vi "Progammable Assembly.vi"   [LabVIEW 2016]
uses:
  Classes/Controller/Controller.lvclass
  Classes/Assembly/Assembly Run.lvclass
  Classes/Routine/Routine Enum.ctl
  Classes/Routine/Routine.lvclass
  Classes/Routine/Settings.ctl
  Classes/Workspace/Fixture Enum.ctl
  Classes/Workspace/Fixture.lvclass
types:
  T1 = typedef "Routine.lvclass/Settings.ctl" = enum16{"Default", "Custom"}
  T2 = typedef "Fixture.lvclass/Fixture Enum.ctl" = enum16{"Assembly Tray", "Syringe Space", "Component", "Pick Up Tool", "Current Position"}
  T3 = typedef "Routine.lvclass/Routine Enum.ctl" = enum16{"Primary Pick Up", "Pick Up All", "Put Down Secondary", "Put Down All", "Release Syringe", "Secondary Pick Up", "Secure Syringe", "Dispense on Plate", "Dispense on Kapton", "Dispense on Sensor"}
  T4 = typedef "Controller.lvclass/Controllers.ctl" = cluster{"I-O.lvclass":refnum<class "I-O.lvclass">, "Motion.lvclass":refnum<class "Motion.lvclass">, "Dispenser.lvclass":refnum<class "Dispenser.lvclass">}
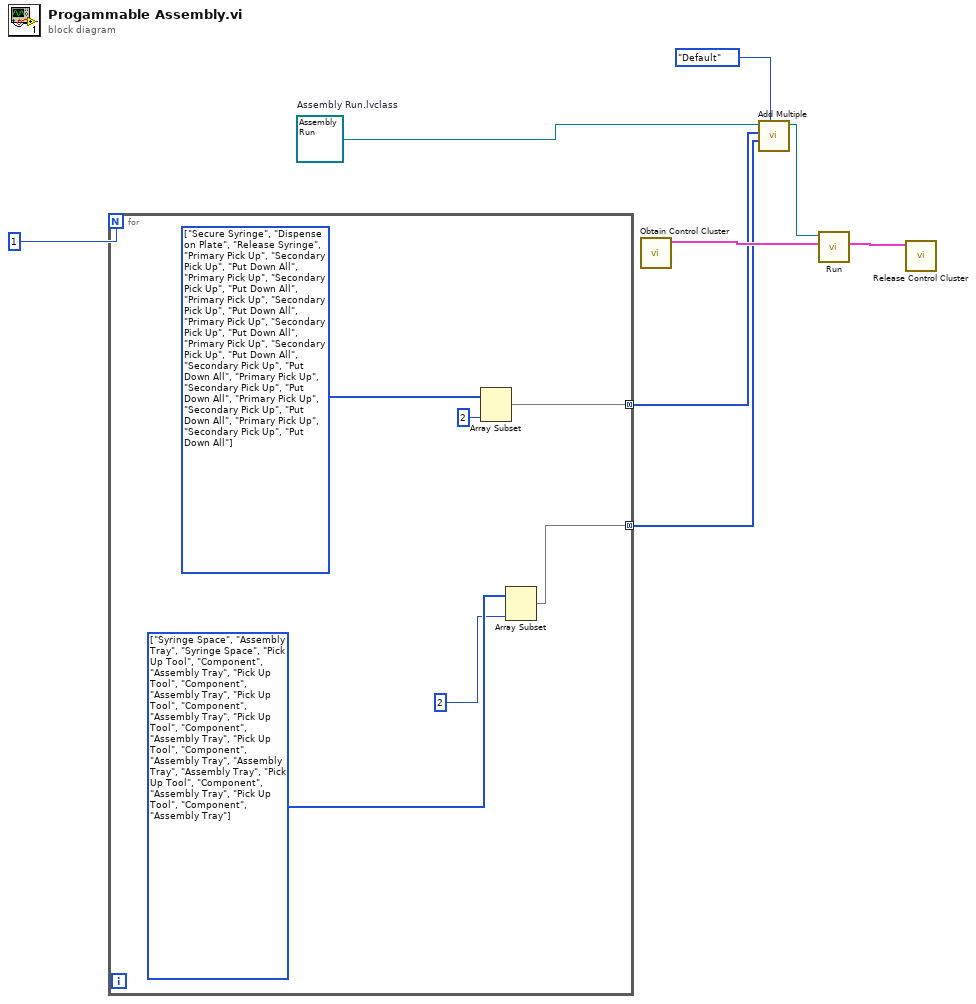
[diagram p0: block diagram]
diagram:
  w1 = refnum<class "Assembly Run.lvclass"> refnum  # Assembly Run.lvclass
  n1 = for {
    N: 1 -> [_]
    tunnel: [w13] -> w5 mode=concatenating
    tunnel: [w10] -> w2 mode=concatenating
    w11 = T2[] [enum."Syringe Space", enum."Assembly Tray", enum."Syringe Space", enum."Pick Up Tool", enum."Component", enum."Assembly Tray", enum."Pick Up Tool", enum."Component", enum."Assembly Tray", enum."Pick Up Tool", enum."Component", enum."Assembly Tray", enum."Pick Up Tool", enum."Component", enum."Assembly Tray", enum."Pick Up Tool", enum."Component", enum."Assembly Tray", enum."Assembly Tray", enum."Assembly Tray", enum."Pick Up Tool", enum."Component", enum."Assembly Tray", enum."Pick Up Tool", enum."Component", enum."Assembly Tray"] items=["Assembly Tray", "Syringe Space", "Component", "Pick Up Tool", "Current Position"]
    w14 = T3[] [enum."Secure Syringe", enum."Dispense on Plate", enum."Release Syringe", enum."Primary Pick Up", enum."Secondary Pick Up", enum."Put Down All", enum."Primary Pick Up", enum."Secondary Pick Up", enum."Put Down All", enum."Primary Pick Up", enum."Secondary Pick Up", enum."Put Down All", enum."Primary Pick Up", enum."Secondary Pick Up", enum."Put Down All", enum."Primary Pick Up", enum."Secondary Pick Up", enum."Put Down All", enum."Secondary Pick Up", enum."Put Down All", enum."Primary Pick Up", enum."Secondary Pick Up", enum."Put Down All", enum."Primary Pick Up", enum."Secondary Pick Up", enum."Put Down All", enum."Primary Pick Up", enum."Secondary Pick Up", enum."Put Down All"] items=["Primary Pick Up", "Pick Up All", "Put Down Secondary", "Put Down All", "Release Syringe", "Secondary Pick Up", "Secure Syringe", "Dispense on Plate", "Dispense on Kapton", "Dispense on Sensor"] ("Routine")
    n2 = Array Subset(array=w14, length=2) -> (w13:T3[])  [unwired: 1 in]
    n3 = Array Subset(array=w11, length=2) -> (w10:T2[])  [unwired: 1 in]
  }
  n4 = call "Obtain Control Cluster.vi"() -> ("Control Out"=w7:T4)  [unwired: 11 in]
  n5 = call-dynamic "Add Multiple.vi"("Settings"=Settings."Default", "Fixtures"=w2, "Routine"=w5, "Assembly in"=w1) -> ("Assembly out"=w8:refnum<class "Assembly Run.lvclass">)  [unwired: 6 in, 1 out]
  n6 = call-dynamic "Run.vi"("Control In"=w7, "Assembly In"=w8) -> ("Control Out"=w6:T4)  [unwired: 7 in, 2 out]
  n7 = call "Release Control Cluster.vi"("output cluster"=w6) -> ()  [unwired: 11 in]
